vi "find input set.vi"(8 "input guess in":i32, 10 "device":u8, 11 "inputs":T1[](array[typedef])) -> (2 "found?":bool, 3 "index out":i32)   [LabVIEW 2013, in "Profibus Module runtime.lvclass"]
uses:
  Profibus Module runtime.lvclass
  profibus slave configuration.ctl
  profibus mapping configuration.ctl
  <vilib>/NI/Tag Bus/tag/Data Type.ctl
  dynamic profibus/full command.ctl
  dynamic profibus/profibus master action.ctl
  <vilib>/NI/Tag Bus/tag/tag descriptor.lvclass
  dynamic profibus/dynamic profibus.lvlib
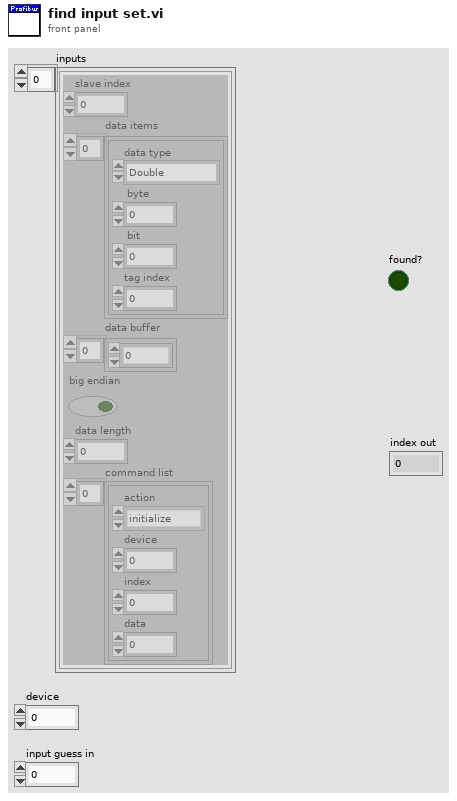
[diagram p1: front panel]
types:
  T1 = typedef "Profibus Module runtime.lvclass/profibus slave configuration.ctl" = cluster{"slave index":i8, "data items":T2[], "data buffer":u8[], "big endian":bool, "data length":i32, "command list":T4[]}
  T2 = typedef "Profibus Module runtime.lvclass/profibus mapping configuration.ctl" = cluster{"data type":T3, " byte":i32, " bit":i32, "tag index":i32}
  T3 = typedef "tag bus.lvlib/tag descriptor.lvclass/Data Type.ctl" = enum16{"Double", "Single", "I64", "I32", "I16", "I8", "U64", "U32", "U16", "U8", "Boolean", "String", "Array of Double", "Array of Single", "Array of I64", "Array of I32", "Array of I16", "Array of I8", "Array of U64", "Array of U32", "Array of U16", "Array of U8", "Array of Boolean", "Array of String"}
  T4 = typedef "dynamic profibus.lvlib/full command.ctl" = cluster{"action":T5, "device":u8, "index":u8, "data":u8}
  T5 = typedef "dynamic profibus.lvlib/profibus master action.ctl" = enum8{"initialize", "uninitialize", "stop", "get input", "get input size", "set output", "get output size", "get diagnostic", "transfer data", "transfer diagnostics"}
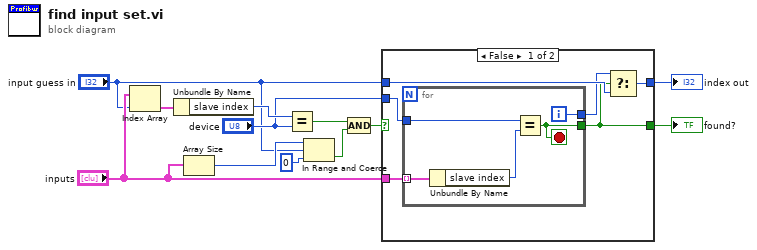
[diagram p0: block diagram]
diagram:
  n1 = Index Array(array="inputs", index="input guess in") -> (element=w11:T1)
  n2 = Unbundle By Name(w11) -> ("slave index"=w10:i8)
  n3 = Array Size(array="inputs") -> (size(s)=w6:i32)
  n4 = Equal?(x=w10, y="device") -> (x = y?=w8:bool)
  n5 = In Range and Coerce(upper limit=w6, x="input guess in", lower limit=0) -> (In Range?=w4:bool)  [unwired: 1 out]
  n6 = Compound Arithmetic op=AND(w8, w4) -> (w3:bool)
  n7 = case shown="False" w3 {
    selector: w3 -> [_ w24]
    tunnel: [w14 w25] -> w12
    tunnel: "device" -> [w18 _]
    tunnel: "input guess in" -> [w16 w25]
    tunnel: "inputs" -> [w17 _]
    tunnel: [w13 w24] -> w2
    frame False {
      n8 = for {
        tunnel: w17 -> [w23] mode=indexing
        tunnel: w18 -> [w21]
        tunnel: [w20] -> w15
        tunnel: [w19] -> w13
        i -> [w20]
        stop <- w19 stop-if-true
        n9 = Unbundle By Name(w23) -> ("slave index"=w22:i8)
        n10 = Equal?(x=w21, y=w22) -> (x = y?=w19:bool)
      }
      n11 = Select(t=w15, s=w13, f=w16) -> (s? t:f=w14:i32)
    }
    frame True {
    }
  }
  "index out" <- w12
  "found?" <- w2
